vi "pumpsec_09_2.vi"(0 "reset":i32, 1 "pump_type":i32, 2 "Target":dbl[](array[numeric])=[10.0, 2.0, 0.0, 0.0, 0.0, 0.0, 0.0, 0.0, 0.0, 0.0], 3 "fr_manual":dbl, 5 "master":i32, 7 "manual":i32, 9 "pause":i32, 11 "Port":i32=10, 12 "port, Reglo D":i32, 14 "Time":dbl[](array[numeric])=[4.0, 2.0, 0.0, 0.0, 0.0, 0.0, 0.0, 0.0, 0.0, 0.0]) -> (4 "Scale":dbl, 6 "mA":dbl format="%#_2g", 8 "Scale actual":dbl, 10 "params":dbl[](array[numeric]), 13 "Reglo D":dbl, 15 "PAM":dbl)   [LabVIEW 2015]
uses:
  BERTTA.dll
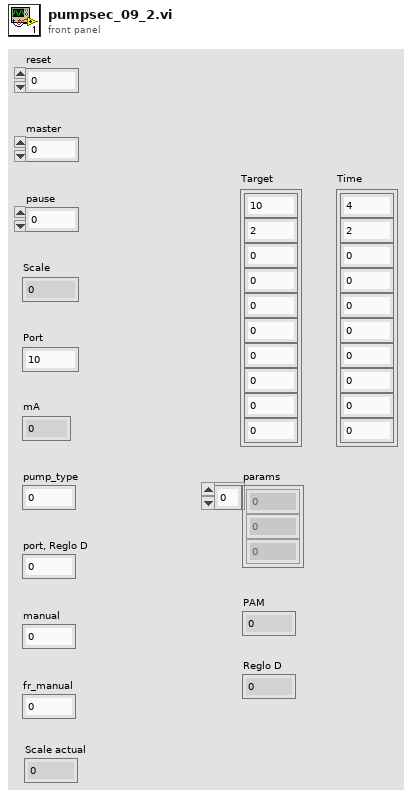
[diagram p1: front panel]
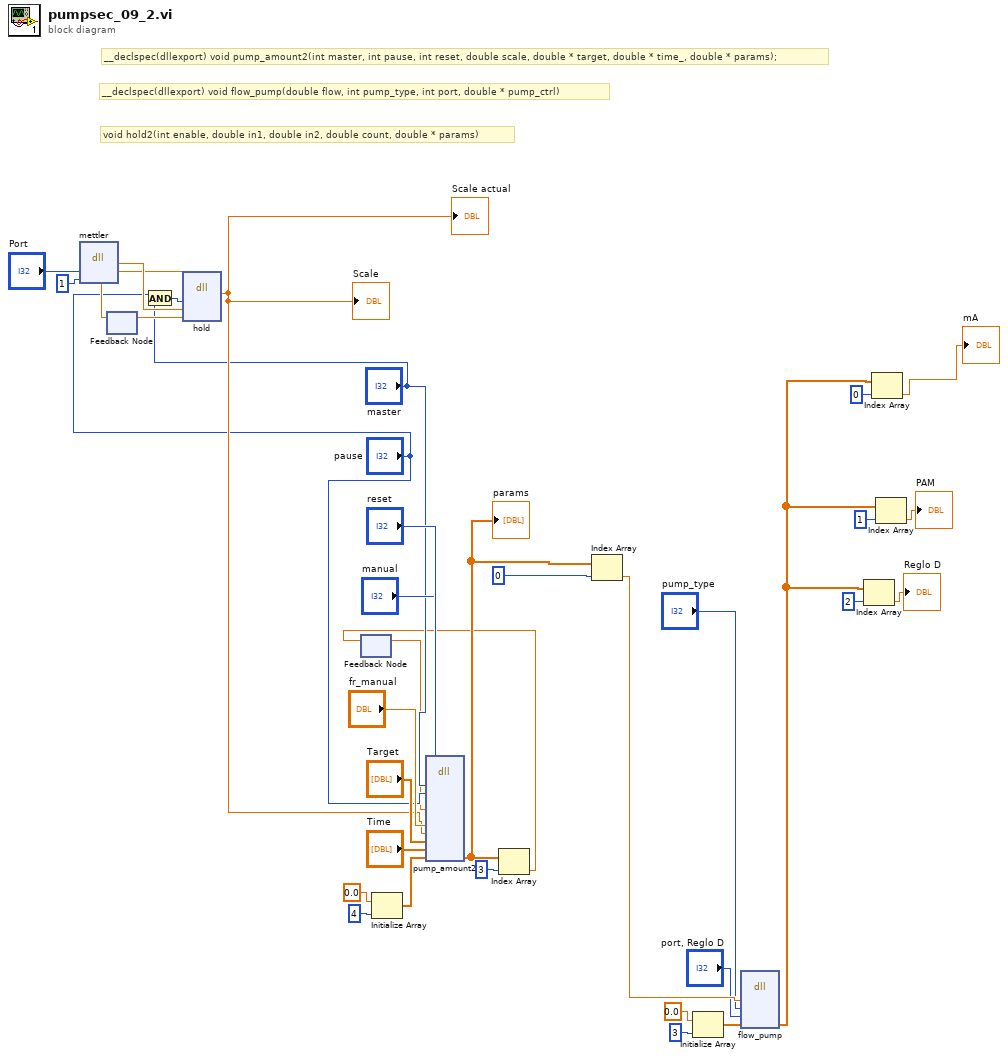
[diagram p0: block diagram]
diagram:
  # "void hold2(int enable, double in1, double in2, double count, double * params)"
  # "__declspec(dllexport) void flow_pump(double flow, int pump_type, int port, double * pump_ctrl)"
  # "__declspec(dllexport) void pump_amount2(int master, int pause, int reset, double scale, double * target, double * time_, double * params);"
  n1 = dll-call lib="C:/Users/shresplab/OneDrive - Kemira Oyj/Documents/Visual Studio 2017/Projects/Bertta/BERTTA/x64/Debug/BERTTA.dll" fn="mettler"("port"="Port", "msg"=1) -> ("return type"=w10:dbl)  [unwired: 5 in, 2 out]
  n2 = feedback #1() -> (w9:dbl)  [unwired: 1 in]
  n3 = And(x="pause", y="master") -> (x .and. y?=w5:i32)
  n4 = dll-call lib="C:/Users/shresplab/OneDrive - Kemira Oyj/Documents/Visual Studio 2017/Projects/Bertta/BERTTA/x64/Debug/BERTTA.dll" fn="hold"("enable"=w5, "in1"=w10, "in2"=w9) -> ("return type"=w8:dbl)  [unwired: 6 in, 2 out]
  "Scale" <- w8
  "Scale actual" <- w8
  n5 = feedback-in #1(w8) -> ()
  n6 = feedback #2() -> (w1:dbl)  [unwired: 1 in]
  n7 = Initialize Array(0.0 ("element"), 4 ("dimension size")) -> (w18:dbl[])
  n8 = dll-call lib="C:/Users/shresplab/OneDrive - Kemira Oyj/Documents/Visual Studio 2017/Projects/Bertta/BERTTA/x64/Debug/BERTTA.dll" fn="pump_amount2"("master"="master", "pause"="pause", "reset"="reset", "count"=w1, "manual"="manual", "fr_manual"="fr_manual", "scale"=w8, "target"="Target", "time_"="Time", "params"=w18) -> ("params"=w3:dbl[])  [unwired: 13 in, 2 out]
  "params" <- w3
  n9 = Index Array(array=w3, index=3) -> (element=w2:dbl)
  n10 = feedback-in #2(w2) -> ()
  n11 = Index Array(array=w3, index=0) -> (element=w28:dbl)
  n12 = Initialize Array(0.0 ("element"), 3 ("dimension size")) -> (w23:dbl[])
  n13 = dll-call lib="C:/Users/shresplab/OneDrive - Kemira Oyj/Documents/Visual Studio 2017/Projects/Bertta/BERTTA/x64/Debug/BERTTA.dll" fn="flow_pump"("flow"=w28, "pump_type"="pump_type", "port"="port, Reglo D", "pump_ctrl"=w23) -> ("pump_ctrl"=w14:dbl[])  [unwired: 7 in, 2 out]
  n14 = Index Array(array=w14, index=2) -> (element=→"Reglo D":dbl)
  n15 = Index Array(array=w14, index=0) -> (element=→"mA":dbl)
  n16 = Index Array(array=w14, index=1) -> (element=→"PAM":dbl)
